vi "Countdown.vi"() -> ()   [LabVIEW 2011]
panel:
  in  "stop":bool
  out "String":string
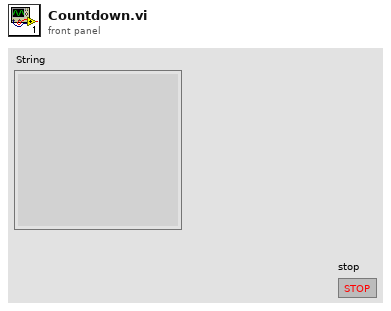
[diagram p1: front panel]
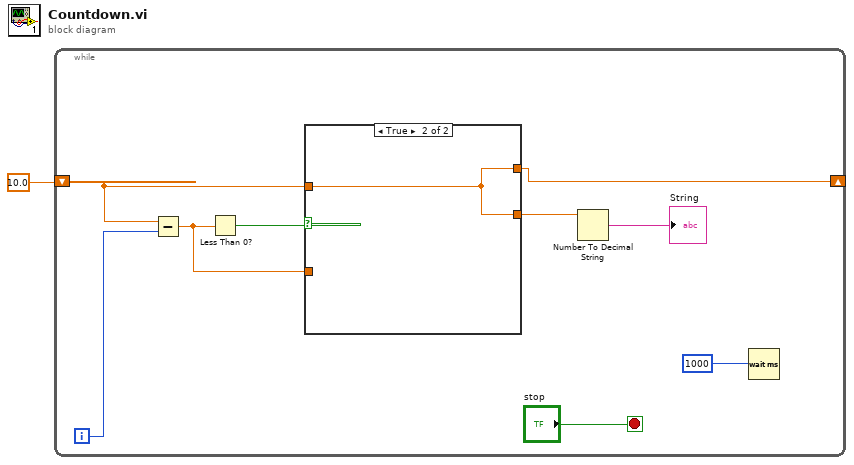
[diagram p0: block diagram]
diagram:
  n1 = while {
    shift-right: [w5] -> _
    shift-left: 10.0 ("x") -> [w2]
    i -> [w10]
    stop <- "stop" stop-if-true
    n2 = Subtract(x=w2, y=w10) -> (x-y=w3:dbl)
    n3 = Less Than 0?(x=w3) -> (x < 0?=w6:bool)
    n4 = case shown="True" w6 {
      tunnel: [w11 w13] -> w5
      tunnel: [w12 w13] -> w4
      tunnel: w3 -> [w12 _]
      tunnel: w2 -> [w11 w13]
      frame False {
      }
      frame True {
      }
    }
    n5 = Number To Decimal String(number=w4) -> (decimal integer string=→"String":string)  [unwired: 1 in]
    n6 = Wait (ms)(milliseconds to wait=u32 1000) -> ()  [unwired: 1 out]
  }
